vi "Read AERs.vi"(8 "error in (no error)":errorcluster, 11 "Cerebellum in":refnum<class "Cerebellum.lvclass">) -> (0 "error out":errorcluster, 1 "AER Right":refnum<class "AER.lvclass">, 2 "AER Left":refnum<class "AER.lvclass">, 3 "Cerebellum out":refnum<class "Cerebellum.lvclass">)   [LabVIEW 2016, in "Cerebellum.lvclass"]
uses:
  Cerebellum.lvclass
  AER/AER.lvclass
  Cerebellum.lvclass/Cerebellum.ctl
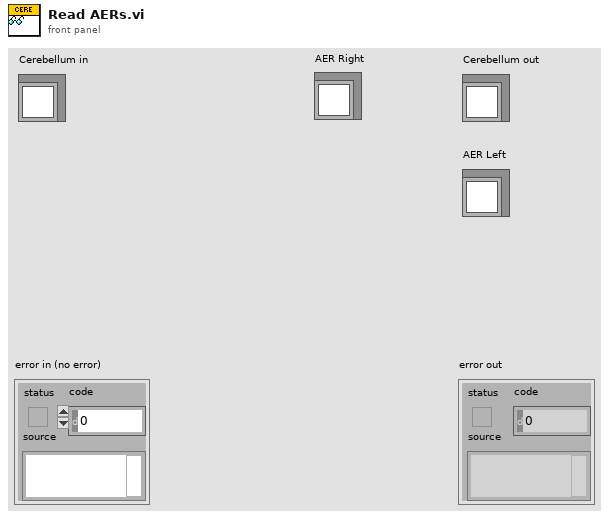
[diagram p1: front panel]
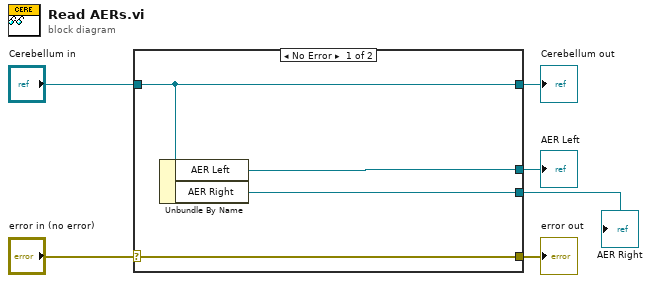
[diagram p0: block diagram]
diagram:
  n1 = case shown="No Error" "error in (no error)" {
    selector: "error in (no error)" -> [w10 w11]
    tunnel: [w10 w11] -> w5
    tunnel: [w9 w12] -> w3
    tunnel: "Cerebellum in" -> [w9 w12]
    tunnel: [w8 _] -> w2
    tunnel: [w7 _] -> w1
    frame No Error {
      n2 = Unbundle By Name(w9) -> ("AER Left"=w8:refnum<class "AER.lvclass">, "AER Right"=w7:refnum<class "AER.lvclass">)
    }
    frame Error {
    }
  }
  "error out" <- w5
  "Cerebellum out" <- w3
  "AER Left" <- w2
  "AER Right" <- w1
